vi "Untitled 1.vi"() -> ()   [LabVIEW 2010]
uses:
  <vilib>/Platform/portaccess.llb/Out Port16.vi
panel:
  in  "Numeric":i16 format="%b"
  in  "address":i16 format="%.0x"
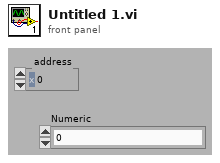
[diagram p1: front panel]
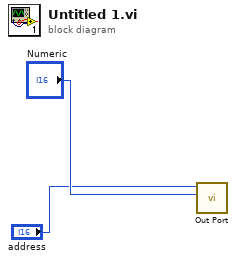
[diagram p0: block diagram]
diagram:
  n1 = call-poly <vilib>:"Out Port.vi"("write value"="Numeric", "address"="address") -> ()  [unwired: 7 in, 1 out]
